vi "SpeedArray.vi"(9 "milliseconds to wait":u32, 11 "Posit Array":T1[](array[typedef])) -> (2 "Speed Array":dbl[](array[numeric]))   [LabVIEW 2014]
uses:
  Libraries/Contact Data/Position.ctl
  Libraries/Contact Data/Contact Data.lvlib
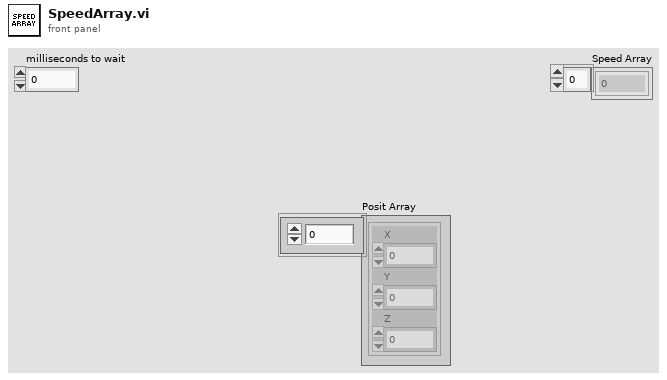
[diagram p1: front panel]
types:
  T1 = typedef "Contact Data.lvlib/Position.ctl" = cluster{"X":dbl, "Y":dbl, "Z":dbl}
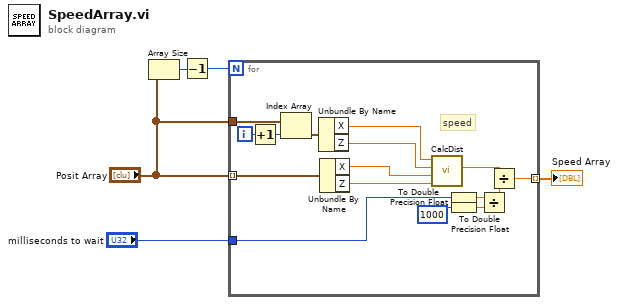
[diagram p0: block diagram]
diagram:
  n1 = Array Size(array="Posit Array") -> (size(s)=w3:i32)
  n2 = Decrement(x=w3) -> (x-1=w2:i32)
  n3 = for {
    N: w2 -> [_]
    tunnel: "Posit Array" -> [w21] mode=indexing
    tunnel: "milliseconds to wait" -> [w8]
    tunnel: "Posit Array" -> [w20]
    tunnel: [w6] -> w1 mode=indexing
    i -> [w19]
    # "speed"
    n4 = Increment(x=w19) -> (x+1=w7:i32)
    n5 = Index Array(array=w20, index=w7) -> (element=w18:T1)
    n6 = Unbundle By Name(w18) -> ("X"=w17:dbl, "Z"=w16:dbl)
    n7 = Unbundle By Name(w21) -> ("X"=w10:dbl, "Z"=w9:dbl)
    n8 = call "CalcDist.vi"("Y2"=w9, "X2"=w10, "Y1"=w16, "X1"=w17) -> ("Distance"=w13:dbl)  [unwired: 7 in]
    n9 = To Double Precision Float(number=w8) -> (double precision float=w12:dbl)
    n10 = To Double Precision Float(number=u32 1000 ("y")) -> (double precision float=w11:dbl)
    n11 = Divide(x=w12, y=w11) -> (x/y=w14:dbl)
    n12 = Divide(x=w13, y=w14) -> (x/y=w6:dbl)
  }
  "Speed Array" <- w1
